vi "Encode ClientID.vi"(10 "Client ID (empty: generate new)":string) -> (2 "valid Client ID":bool, 3 "Length-Prefixed Field":u8[](array[numeric]) format="%08b")   [LabVIEW 2013, in "ControlPacket.lvclass"]
uses:
  ControlPacket.lvclass
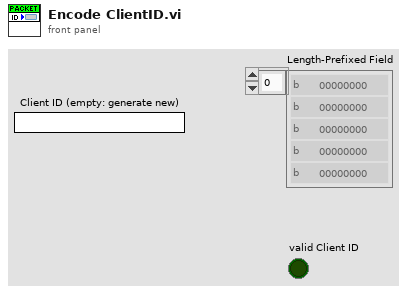
[diagram p1: front panel]
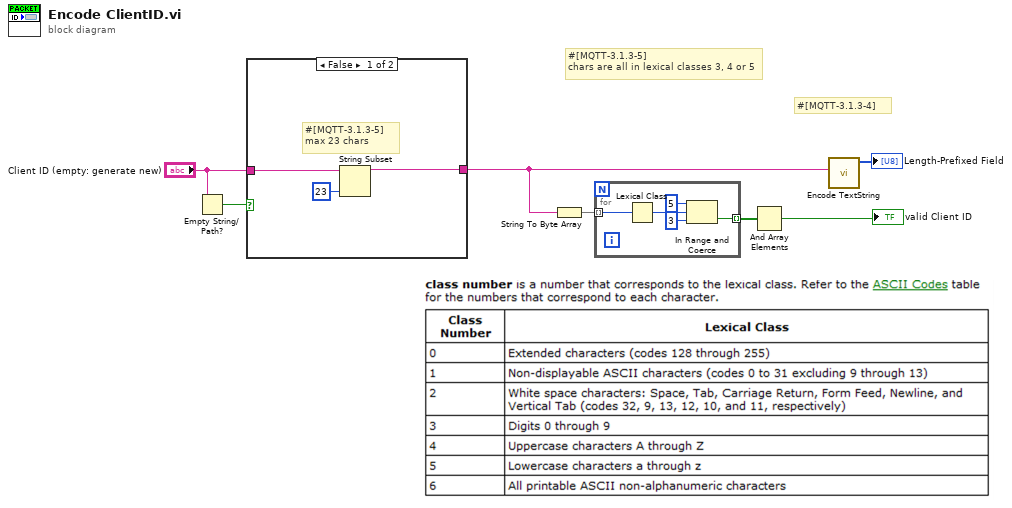
[diagram p0: block diagram]
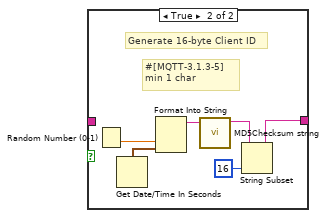
[diagram p2: hidden frame]
diagram:
  # "#[MQTT-3.1.3-5]\nchars are all in lexical classes 3, 4 or 5"
  # "#[MQTT-3.1.3-4]"
  n1 = Empty String/Path?(string/path="Client ID (empty: generate new)") -> (empty?=w7:bool)
  n2 = case shown="False" w7 {
    tunnel: "Client ID (empty: generate new)" -> [w9 _]
    tunnel: [w8 w11] -> w4
    frame False {
      # "#[MQTT-3.1.3-5]\nmax 23 chars"
      n3 = String Subset(string=w9, length (rest)=23 ("length (rest)")) -> (substring=w8:string)  [unwired: 1 in]
    }
    frame True {
      # "#[MQTT-3.1.3-5]\nmin 1 char"
      # "Generate 16-byte Client ID"
      n4 = Random Number (0-1)() -> (number: 0 to 1=w15:dbl)
      n5 = Get Date/Time In Seconds() -> (seconds since 1Jan1904=w14:timestamp)
      n6 = Format Into String(w15, w14) -> (resulting string=w16:string)  [unwired: 3 in, 1 out]
      n7 = call <vilib>:"MD5Checksum string.vi"("Message String"=w16) -> ("MD5 message-digest"=w13:string)  [unwired: 10 in]
      n8 = String Subset(string=w13, length (rest)=16 ("length (rest)")) -> (substring=w11:string)  [unwired: 1 in]
    }
  }
  n9 = String To Byte Array(string=w4) -> (unsigned byte array=w1:u8[])
  n10 = for {
    tunnel: w1 -> [w21] mode=indexing
    tunnel: [w17] -> w3 mode=indexing
    n11 = Lexical Class(1:w21) -> (0:w20:i16)
    n12 = In Range and Coerce(upper limit=i16 5, x=w20, lower limit=i16 3) -> (In Range?=w17:bool)  [unwired: 1 out]
  }
  n13 = And Array Elements(Boolean array=w3) -> (logical AND=→"valid Client ID":bool)
  n14 = call "Encode TextString.vi"("Text String"=w4) -> ("Length-Prefixed Field"=→"Length-Prefixed Field":u8[])  [unwired: 10 in]
